vi "PH_BeamlineController.set Target GUI Elements.vi"(0 "VI in":refnum<vi>, 5 "error in (no error)":errorcluster) -> (14 "VI out":refnum<vi>, 19 "error out":errorcluster)   [LabVIEW 2014, in "PH_BeamlineController.lvlib"]
uses:
  PH_BeamlineController.lvlib
  PH_SystemInformation/PH_SystemInformationEnabling State.ctl
  PH_BeamlineController.Sources.ctl
  PH_BeamlineController.PA DP Targets.ctl
  PH_StatusHandler/PH_StatusHandler.Status.ctl
  PH_SystemInformation/PH_SystemInformation.lvlib
  PH_StatusHandler/PH_StatusHandler.lvlib
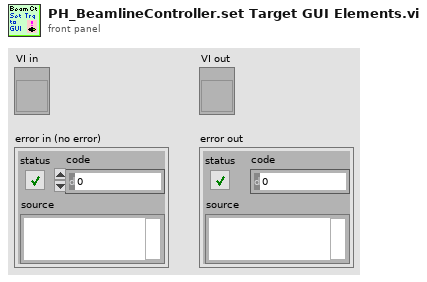
[diagram p1: front panel]
types:
  T1 = typedef "PH_BeamlineController.lvlib/PH_BeamlineController.PA DP Targets.ctl" = enum16{"None", "Dump PA Delayed Beam", "Dump PA Undelayed Beam", "Dumps PA Delayed and Undelayed Beam"}
  T2 = typedef "PH_SystemInformation.lvlib/PH_SystemInformationEnabling State.ctl" = i32
  T3 = enum16{"Laser", "PreAmp", "MainAmp", "Exp 1", "Exp 2", "Exp 3", "Exp 4"}
  T4 = typedef "PH_BeamlineController.lvlib/PH_BeamlineController.Sources.ctl" = enum16{"None", "YLF", "fs-Frontend", "ns-Frontend", "YLF and ns-Frontend", "fs- and ns-Frontend"}
  T5 = enum8{"Enabled", "Disabled", "Disabled and Grayed Out"}
  T6 = typedef "PH_StatusHandler.lvlib/PH_StatusHandler.Status.ctl" = i16
  T7 = typedef "PH_BeamlineController.lvlib/PH_BeamlineController.i attribute.ctl" = cluster{"Vacuum Exp LB":cluster{"Channel":string, "Limit [mbar]":dbl, "Pressure [mbar]":dbl, "GUI Ref":refnum<vi>}, "Sources":T8[], "PA DP Targets":T9[], "Path":cluster{"Source":T4, "PA DP Target":T1, "Target":T10}, "Targets":cluster{"Name":T10, "GUI Ref":refnum<vi>, "Current State":bool, "Wanted State":bool, "Enabled":bool}[], "Status Tags":cluster{"Name":string, "Status":T6}[], "special GUI Refs":T11}
  T8 = typedef "PH_BeamlineController.lvlib/PH_BeamlineController.Source Attributes.ctl" = cluster{"Name":T4, "GUI Ref":refnum<vi>, "Current State":bool, "Wanted State":bool}
  T9 = typedef "PH_BeamlineController.lvlib/PH_BeamlineController.PA DP Target Attributes.ctl" = cluster{"Name":T1, "GUI Ref":refnum<vi>, "Current State":bool, "Wanted State":bool, "Enabled":bool}
  T10 = typedef "PH_BeamlineController.lvlib/PH_BeamlineController.Targets.ctl" = enum16{"None", "PreAmp", "Dump Exp Laserlab", "Exp Laserlab", "Calorimeter", "Dump Exp Laserbay", "Exp Laserbay", "Dump Exp Z6", "Exp Z6"}
  T11 = typedef "PH_BeamlineController.lvlib/PH_BeamlineController.special GUI Refs.ctl" = cluster{"PA-Backreflection-Meas":refnum<vi>, "fs_Synchrolock_Watch":refnum<vi>}
  T12 = cluster{"Name":T10, "GUI Ref":refnum<vi>, "Current State":bool, "Wanted State":bool, "Enabled":bool}[]
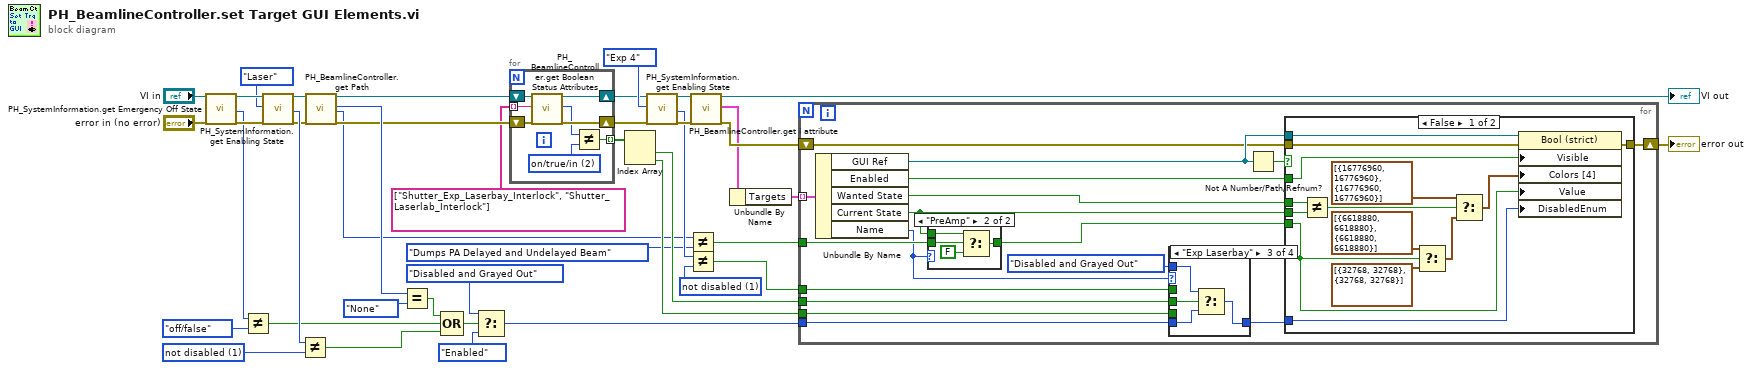
[diagram p0: block diagram]
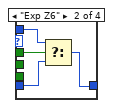
[diagram p4: hidden frame]
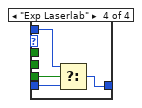
[diagram p5: hidden frame]
diagram:
  w15 = T2 1 items=["no info", "not disabled", "disabled"] ("y")
  w33 = T2 1 items=["no info", "not disabled", "disabled"] ("y")
  n1 = call "PH_SystemInformation.get Emergency Off State.vi"("i ref in"="VI in", "error in (no error)"="error in (no error)") -> ("i ref out"=w39:refnum<vi>, "Emergency Off State"=w36:enum16{"no info", "off/false", "Alarm"}, "error out"=w38:errorcluster)  [unwired: 15 in]
  n2 = Not Equal?(x=w36, y=enum16{"no info", "off/false", "Alarm"}."off/false") -> (x != y?=w23:bool)
  n3 = call "PH_SystemInformation.get Enabling State.vi"("i ref in"=w39, "Wanted State"=T3."Laser", "error in (no error)"=w38) -> ("i ref out"=w26:refnum<vi>, "Enabling State"=w34:T2, "error out"=w25:errorcluster)  [unwired: 14 in]
  n4 = Not Equal?(x=w34, y=w33) -> (x != y?=w24:bool)
  n5 = call "PH_BeamlineController.get Path.vi"("VI in"=w26, "error in (no error)"=w25) -> ("VI out"=w9:refnum<vi>, "Path: Source"=w20:T4, "Path:  PA DP Targets"=w3:T1, "error out"=w18:errorcluster)  [unwired: 12 in, 2 out]
  n6 = Equal?(x=w20, y=PH_BeamlineController.Sources."None" ("Source")) -> (x = y?=w21:bool)
  n7 = Compound Arithmetic op=OR(w21, w23, w24) -> (w22:bool)
  n8 = Select(t=T5."Disabled and Grayed Out" ("Disabled"), s=w22, f=T5."Enabled" ("Disabled")) -> (s? t:f=w28:T5)
  n9 = for {
    shift-right: [w49] -> w10
    shift-left: w18 -> [w50]
    shift-right: [w47] -> w8
    shift-left: w9 -> [w48]
    tunnel: string[] ["Shutter_Exp_Laserbay_Interlock", "Shutter_Laserlab_Interlock"] -> [w46] mode=indexing
    tunnel: [w43] -> w6 mode=indexing
    w44 = T6 2 items=["no info", "off/false/out", "on/true/in", "Failure", "Alarm", "Status 1", "Status 2", "Status 3"] ("y")
    n10 = call "PH_BeamlineController.get Boolean Status Attributes.vi"("VI in"=w48, "Name"=w46, "error in (no error)"=w50) -> ("VI out"=w47:refnum<vi>, "Status"=w45:T6, "error out"=w49:errorcluster)  [unwired: 11 in, 3 out]
    n11 = Not Equal?(x=w45, y=w44) -> (x != y?=w43:bool)
  }
  n12 = Index Array(array=w6) -> (element #1=w4:bool, element #2=w5:bool)  [unwired: 2 in]
  n13 = call "PH_SystemInformation.get Enabling State.vi"("i ref in"=w8, "Wanted State"=T3."Exp 4", "error in (no error)"=w10) -> ("i ref out"=w19:refnum<vi>, "Enabling State"=w14:T2, "error out"=w17:errorcluster)  [unwired: 14 in]
  n14 = Not Equal?(x=w3, y=PH_BeamlineController.PA_DP_Targets."Dumps PA Delayed and Undelayed Beam") -> (x != y?=w1:bool)
  n15 = Not Equal?(x=w14, y=w15) -> (x != y?=w13:bool)
  n16 = call "PH_BeamlineController.get i attribute.vi"("i ref in"=w19, "error in (no error)"=w17) -> ("i ref out"=→"VI out":refnum<vi>, "i attribute"=w41:T7, "error out"=w42:errorcluster)  [unwired: 15 in]
  n17 = Unbundle By Name(w41) -> ("Targets"=w40:T12)
  n18 = for {
    shift-right: [w67] -> w11
    shift-left: w42 -> [w61]
    tunnel: w40 -> [w66] mode=indexing
    tunnel: w28 -> [w59]
    tunnel: w13 -> [w60]
    tunnel: w5 -> [w56]
    tunnel: w4 -> [w55]
    tunnel: w1 -> [w54]
    n19 = Unbundle By Name(w66) -> ("GUI Ref"=w64:refnum<vi>, "Enabled"=w62:bool, "Wanted State"=w65:bool, "Current State"=w53:bool, "Name"=w51:T10)
    n20 = case shown="\"PreAmp\"" w51 {
      tunnel: w54 -> [_ w72]
      tunnel: w53 -> [w68 w71]
      tunnel: [w68 w70] -> w52
      frame Default {
      }
      frame "PreAmp" {
        n21 = Select(t=w71, s=w72, f=FALSE) -> (s? t:f=w70:bool)
      }
    }
    n22 = case shown="\"Exp Laserbay\"" w51 {
      tunnel: w60 -> [_ w77 _ _]
      tunnel: w59 -> [w73 w76 w81 w85]
      tunnel: [w73 w75 w80 w84] -> w58
      tunnel: T5."Disabled and Grayed Out" ("Disabled") -> [_ w74 w79 w83]
      tunnel: w56 -> [_ _ _ w82]
      tunnel: w55 -> [_ _ w78 _]
      frame Default {
      }
      frame "Exp Z6" {
        n23 = Select(t=w74, s=w77, f=w76) -> (s? t:f=w75:T5)
      }
      frame "Exp Laserbay" {
        n24 = Select(t=w79, s=w78, f=w81) -> (s? t:f=w80:T5)
      }
      frame "Exp Laserlab" {
        n25 = Select(t=w83, s=w82, f=w85) -> (s? t:f=w84:T5)
      }
    }
    n26 = Not A Number/Path/Refnum?(number/path/refnum=w64) -> (NaN/Path/Refnum?=w63:bool)
    n27 = case shown="False" w63 {
      tunnel: w61 -> [w99 w100]
      tunnel: [w98 w100] -> w67
      tunnel: w64 -> [w97 _]
      tunnel: w65 -> [w91 _]
      tunnel: w53 -> [w90 _]
      tunnel: w58 -> [w89 _]
      tunnel: w62 -> [w87 _]
      tunnel: w52 -> [w86 _]
      frame False {
        n28 = Not Equal?(x=w91, y=w90) -> (x != y?=w94:bool)
        n29 = Select(t=cluster{"Color Box":u32, "Color Box 2":u32}[] [{"Color Box"=6618880, "Color Box 2"=6618880}, {"Color Box"=6618880, "Color Box 2"=6618880}], s=w86, f=cluster{"Color Box":u32, "Color Box 2":u32}[] [{"Color Box"=32768, "Color Box 2"=32768}, {"Color Box"=32768, "Color Box 2"=32768}]) -> (s? t:f=w92:cluster{"Color Box":u32, "Color Box 2":u32}[])
        n30 = Select(t=cluster{"Color Box":u32, "Color Box 2":u32}[] [{"Color Box"=16776960, "Color Box 2"=16776960}, {"Color Box"=16776960, "Color Box 2"=16776960}], s=w94, f=w92) -> (s? t:f=w88:cluster{"Color Box":u32, "Color Box 2":u32}[])
        n31 = property class="Bool (strict)"(reference=w97, error in=w99, "Visible"=w87, "Colors [4]"=w88, "Value"=w86, "DisabledEnum"=w89) -> (error out=w98:errorcluster)  [unwired: 1 out]
      }
      frame True {
      }
    }
  }
  "error out" <- w11
